vi "Read To String Delimiter.vi"(8 "error in (no error)":errorcluster, 11 "Abs_Double Float 1D in":refnum<class "Abs_U64 Integer 1D.lvclass">) -> (0 "error out":errorcluster, 2 "Delimiter":string, 3 "Abs_Double Float 1D out":refnum<class "Abs_U64 Integer 1D.lvclass">)   [LabVIEW 2019]
uses:
  Abs_U64 Integer 1D.lvclass
  Abs_U64 Integer 1D.lvclass/Abs_U64 Integer 1D.ctl
  C:/TSA/LV_Abstract_2019/TSA/LV_Abstract/Source/Abs_Types/Integer 1D/Abs_Integer 1D.lvclass
  C:/TSA/LV_Abstract_2019/TSA/LV_Abstract/Source/Abs_Types/Numeric 1D/Abs_Numeric_1D.lvclass
  C:/TSA/LV_Abstract_2019/TSA/LV_Abstract/Source/Abs_Types/Value/Abs_Value.lvclass
  C:/TSA/LV_Abstract_2019/TSA/LV_Abstract/Source/Abs_Types/Type/Abs_Type.lvclass
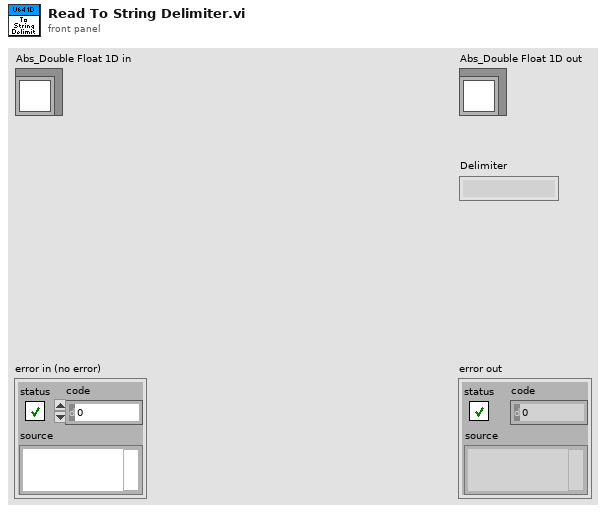
[diagram p1: front panel]
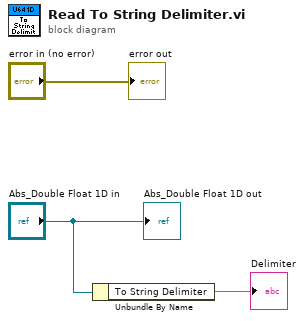
[diagram p0: block diagram]
diagram:
  n1 = Unbundle By Name("Abs_Double Float 1D in") -> ("To String Delimiter"=→"Delimiter")
  "error out" <- "error in (no error)"
  "Abs_Double Float 1D out" <- "Abs_Double Float 1D in"
